vi "Drive Ramp.vi"(8 "Max Delta Per Iteration":dbl=0.2, 11 "Input":dbl) -> (3 "Output":dbl)   [LabVIEW 2013]
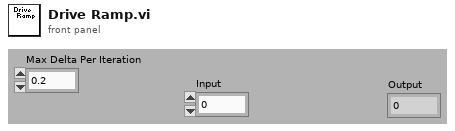
[diagram p1: front panel]
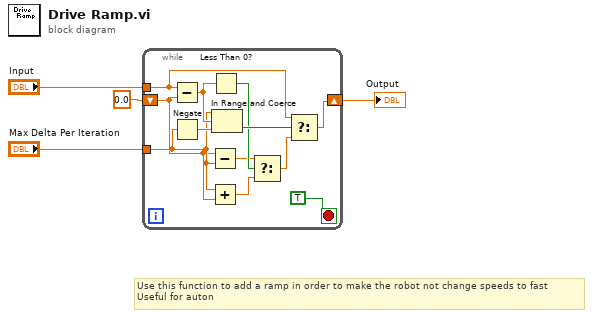
[diagram p0: block diagram]
diagram:
  # "Use this function to add a ramp in order to make the robot not change speeds to fast\nUseful for auton"
  n1 = while {
    shift-right: [w12] -> w1
    shift-left: 0.0 -> [w5]
    tunnel: "Max Delta Per Iteration" -> [w6]
    tunnel: "Input" -> [w13]
    stop <- TRUE stop-if-true
    n2 = Subtract(x=w13, y=w5) -> (x-y=w11:dbl)
    n3 = Negate(x=w6) -> (-x=w15:dbl)
    n4 = Subtract(x=w5, y=w6) -> (x-y=w8:dbl)
    n5 = Add(x=w6, y=w5) -> (x+y=w7:dbl)
    n6 = Less Than 0?(x=w11) -> (x < 0?=w9:bool)
    n7 = In Range and Coerce(upper limit=w6, x=w11, lower limit=w15) -> (In Range?=w14:bool)  [unwired: 1 out]
    n8 = Select(t=w8, s=w9, f=w7) -> (s? t:f=w10:dbl)
    n9 = Select(t=w13, s=w14, f=w10) -> (s? t:f=w12:dbl)
  }
  "Output" <- w1
